vi "原始值线性转换.vi"(7 "AD线性关系":T2(array[cluster])=[{"X0"=1638.0, "X1"=8191.0, "Y0"=-40.0, "Y1"=100.0}, {"X0"=1638.0, "X1"=8191.0, "Y0"=0.0, "Y1"=100.0}, {"X0"=1638.0, "X1"=8191.0, "Y0"=0.0, "Y1"=1.0}, {"X0"=0.0, "X1"=8191.0, "Y0"=0.0, "Y1"=8191.0}, {"X0"=0.0, "X1"=8191.0, "Y0"=0.0, "Y1"=8191.0}, {"X0"=0.0, "X1"=8191.0, "Y0"=0.0, "Y1"=8191.0}, {"X0"=0.0, "X1"=8191.0, "Y0"=0.0, "Y1"=8191.0}, {"X0"=0.0, "X1"=8191.0, "Y0"=0.0, "Y1"=8191.0}], 11 "AD当前原始值":T3 {"AD7" format="%.2f"; "AD6" format="%.2f"; "AD5" format="%.2f"; "AD4" format="%.2f"; "AD3" format="%.2f"; "AD1" format="%.2f"; "AD1" format="%.2f"; "AD0" format="%.2f"}) -> (3 "AD当前转换值":T1 {"AD7" format="%.2f"; "AD6" format="%.2f"; "AD5" format="%.2f"; "AD4" format="%.2f"; "AD3" format="%.2f"; "AD2" format="%.2f"; "AD1" format="%.2f"; "AD0" format="%.2f"})   [LabVIEW 2016, in "环境动力监测库.lvlib"]
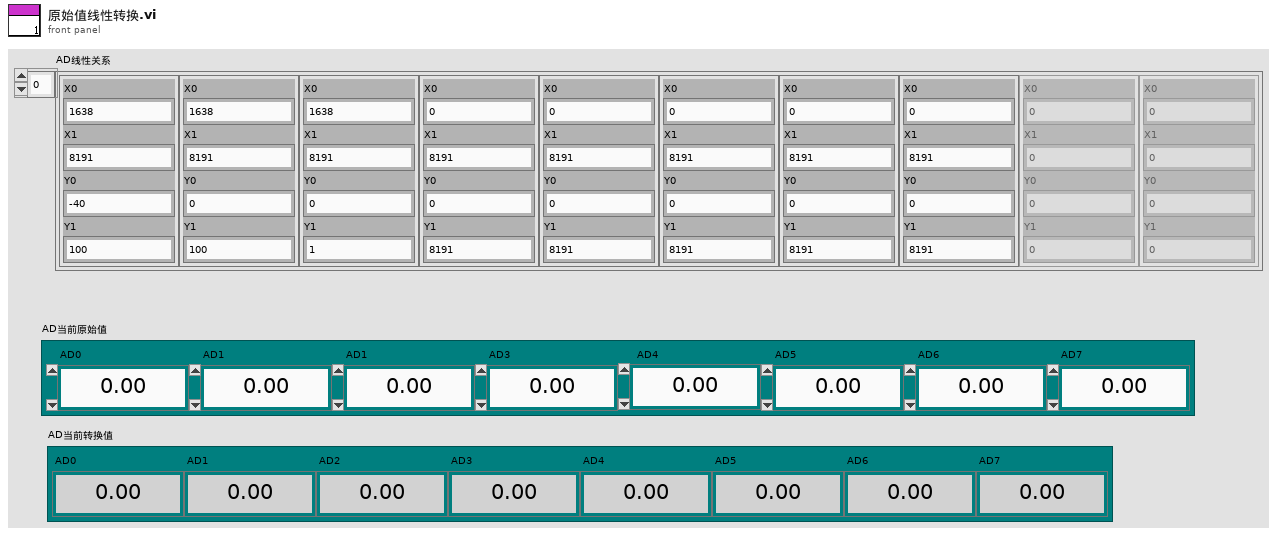
[diagram p1: front panel]
types:
  T1 = cluster{"AD0":dbl, "AD1":dbl, "AD2":dbl, "AD3":dbl, "AD4":dbl, "AD5":dbl, "AD6":dbl, "AD7":dbl}
  T2 = cluster{"X0":dbl, "X1":dbl, "Y0":dbl, "Y1":dbl}[]
  T3 = cluster{"AD0":dbl, "AD1":dbl, "AD1":dbl, "AD3":dbl, "AD4":dbl, "AD5":dbl, "AD6":dbl, "AD7":dbl}
  T4 = cluster{"[0]":dbl, "[1]":dbl, "[2]":dbl, "[3]":dbl, "[4]":dbl, "[5]":dbl, "[6]":dbl, "[7]":dbl}
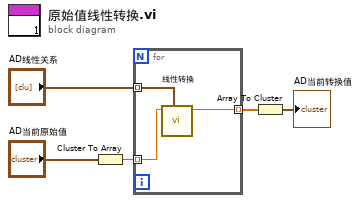
[diagram p0: block diagram]
diagram:
  n1 = Cluster To Array(cluster="AD当前原始值") -> (array=w4:dbl[])
  n2 = for {
    tunnel: w4 -> [w8] mode=indexing
    tunnel: "AD线性关系" -> [w7] mode=indexing
    tunnel: [w6] -> w2 mode=indexing
    n3 = call "线性转换.vi"("线性关系"=w7, "input"=w8) -> ("output"=w6:dbl)  [unwired: 9 in]
  }
  n4 = Array To Cluster(array=w2) -> (cluster=→"AD当前转换值":T4)
